vi "InitSnakes.vi"(8 "error in (no error)":errorcluster, 11 "SnakeDemo in":refnum<class "SnakeDemo.lvclass">) -> (0 "error out":errorcluster, 3 "SnakeDemo out":refnum<class "SnakeDemo.lvclass">)   [LabVIEW 2019, in "RT_Game.lvlib" / "SnakeDemo.lvclass"]
uses:
  SnakeDemo.lvclass
  C:/Users/FreshBob/Dropbox/VIs/myRIO_GameConsole/RT/RT_Game/SnakeGame/SnakeGame.lvclass
  AI_Snake/AI_Snake.lvclass
  C:/Users/FreshBob/Dropbox/VIs/myRIO_GameConsole/RT/RT_Game/Snake/Snake.lvclass
  Snake/Snake.lvclass
  Snake/CoordinateData.ctl
  Game/Coordinate.ctl
  Snake/Direction.ctl
  Snake/Snake.lvclass/Snake.ctl
  SnakeGame/SnakeGame.lvclass/SnakeGame.ctl
  Snake/Write Dead_.vi
  Snake/Write Color.vi
  Snake/Write Coordinates.vi
  Snake/Write Direction.vi
  Snake/Write ScorePosition.vi
  Snake/Write tick_rate.vi
  Snake/Write Length.vi
  Snake/Write speed_multiplier.vi
  Snake/Write DoTick.vi
  SnakeGame/Write Snakes.vi
  Game/Game.lvclass
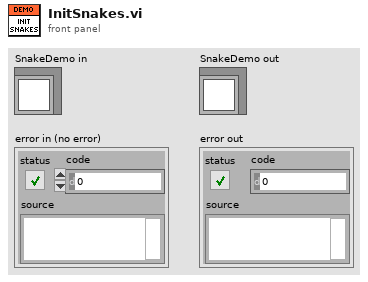
[diagram p1: front panel]
types:
  T1 = typedef "RT_Game.lvlib/Game.lvclass/Coordinate.ctl" = cluster{"x":dbl, "y":dbl}
  T2 = typedef "RT_Game.lvlib/Snake.lvclass/Direction.ctl" = enum16{"Up", "Left", "Down", "Right"}
  T3 = typedef "RT_Game.lvlib/Snake.lvclass/CoordinateData.ctl" = cluster{"Coordinate":T1, "TileCode":u32}
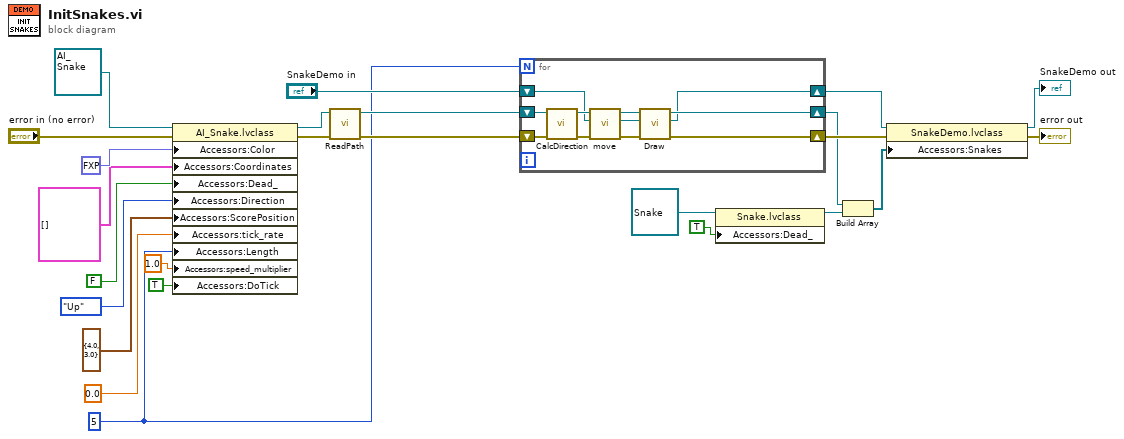
[diagram p0: block diagram]
diagram:
  w2 = i16 5 ("Length")
  n1 = property class="AI_Snake.lvclass"(reference=refnum<class "AI_Snake.lvclass"> refnum ("RT_Game.lvlib:AI_Snake.lvclass"), error in="error in (no error)", "Accessors:Color"=fxp<+,3,3> 4.0 ("Color"), "Accessors:Coordinates"=T3[] [] ("Coordinates"), "Accessors:Dead_"=FALSE ("Dead_"), "Accessors:Direction"=Direction."Up" ("Direction"), "Accessors:ScorePosition"=T1 {"x"=4.0, "y"=3.0} ("ScorePosition"), "Accessors:tick_rate"=0.0 ("tick_rate"), "Accessors:Length"=w2, "Accessors:speed_multiplier"=1.0 ("speed_multiplier"), "Accessors:DoTick"=TRUE ("DoTick")) -> (reference out=w12:refnum<class "AI_Snake.lvclass">, error out=w14:errorcluster)
  n2 = call "ReadPath.vi"("error in (no error)"=w14, "AI_Snake in"=w12) -> ("error out"=w18:errorcluster, "AI_Snake out"=w4:refnum<class "AI_Snake.lvclass">)  [unwired: 8 in]
  n3 = for {
    N: w2 -> [_]
    shift-right: [w30] -> w17
    shift-left: w18 -> [w36]
    shift-right: [w28] -> w16
    shift-left: w4 -> [w33]
    shift-right: [w26] -> w15
    shift-left: "SnakeDemo in" -> [w31]
    n4 = call "CalcDirection.vi"("error in (no error)"=w36, "Snake in"=w33) -> ("error out"=w34:errorcluster, "Snake out"=w32:refnum<class "AI_Snake.lvclass">)  [unwired: 8 in]
    n5 = call "move.vi"("error in (no error)"=w34, "SnakeGame in"=w31, "Snake in"=w32) -> ("error out"=w35:errorcluster, "SnakeGame out"=w27:refnum<class "SnakeDemo.lvclass">, "Snake out"=w29:refnum<class "AI_Snake.lvclass">)  [unwired: 6 in]
    n6 = call "Draw.vi"("error in (no error)"=w35, "Snake in 2"=w27, "Snake in"=w29) -> ("error out"=w30:errorcluster, "Snake out 2"=w26:refnum<class "SnakeDemo.lvclass">, "Snake out"=w28:refnum<class "AI_Snake.lvclass">)  [unwired: 6 in]
  }
  n7 = property class="Snake.lvclass"(reference=refnum<class "Snake.lvclass"> refnum ("RT_Game.lvlib:Snake.lvclass"), "Accessors:Dead_"=TRUE ("Dead_")) -> (reference out=w21:refnum<class "Snake.lvclass">)  [unwired: 1 in, 1 out]
  n8 = Build Array(w16, w21) -> (w20:refnum<class "Snake.lvclass">[])
  n9 = property class="SnakeDemo.lvclass"(reference=w15, error in=w17, "Accessors:Snakes"=w20) -> (reference out=→"SnakeDemo out":refnum<class "SnakeDemo.lvclass">, error out=→"error out":errorcluster)
